vi "error_handle_EoF.vi"(8 "error in":errorcluster, 11 "Remove EoF Error?":bool) -> (0 "error out":errorcluster, 2 "specific error cleared?":bool, 3 "is EoF?":bool)   [LabVIEW 2016]
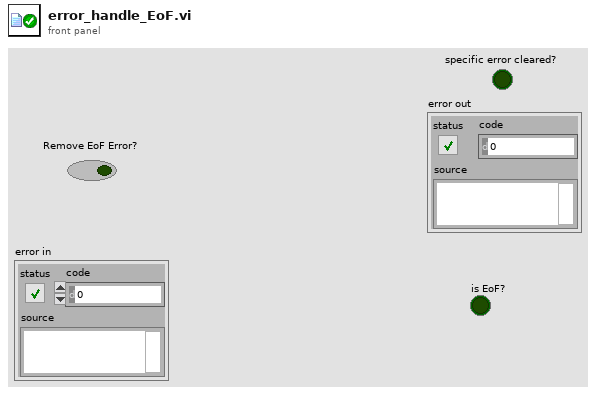
[diagram p1: front panel]
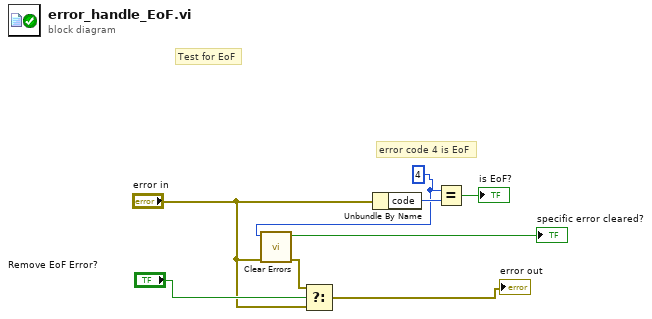
[diagram p0: block diagram]
diagram:
  w4 = 4 ("x")
  # "Test for EoF"
  # "error code 4 is EoF"
  n1 = call <vilib>:"Clear Errors.vi"("error in (no error)"="error in", "specific error code to clear (0: all)"=w4) -> ("error out"=w3:errorcluster, "specific error cleared?"=→"specific error cleared?":bool)  [unwired: 4 in]
  n2 = Select(t=w3, s="Remove EoF Error?", f="error in") -> (s? t:f=→"error out":errorcluster)
  n3 = Unbundle By Name("error in") -> ("code"=w8:i32)
  n4 = Equal?(x=w4, y=w8) -> (x = y?=→"is EoF?":bool)
